vi "Velocity In Range.vi"(8 "Velocity Tolerance":dbl, 9 "Target Velocity":dbl, 10 "Current Velocity":dbl) -> (1 "In Range?":bool)   [LabVIEW 2017]
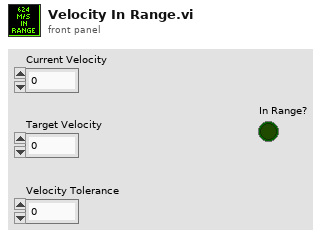
[diagram p1: front panel]
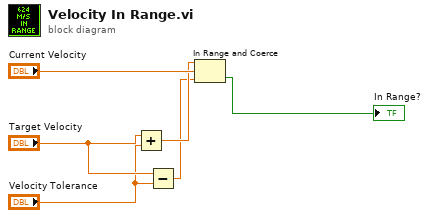
[diagram p0: block diagram]
diagram:
  n1 = Add(x="Target Velocity", y="Velocity Tolerance") -> (x+y=w5:dbl)
  n2 = Subtract(x="Target Velocity", y="Velocity Tolerance") -> (x-y=w2:dbl)
  n3 = In Range and Coerce(upper limit=w5, x="Current Velocity", lower limit=w2) -> (In Range?=→"In Range?":bool)  [unwired: 1 out]
